vi "Utility MODBUS RTU CRC16.vi"(8 "error in (no error)":errorcluster, 10 "Message (empty array)":u8[](array[numeric]) format="%.0x", 11 "VISA resource name":refnum<visa-resource-name>) -> (0 "error out":errorcluster, 1 "CRC":u16 format="%.0x", 2 "Message with CRC":u8[](array[numeric]) format="%.0x", 3 "VISA resource name out":refnum<visa-resource-name>)   [LabVIEW 2010]
doc: "This VI computes the CRC code and appends it to the message."
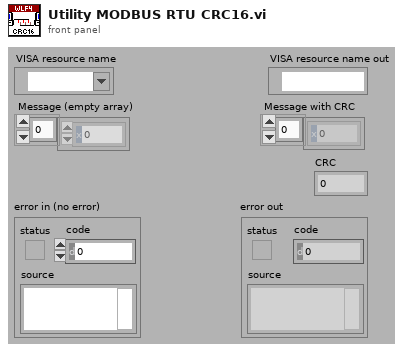
[diagram p1: front panel]
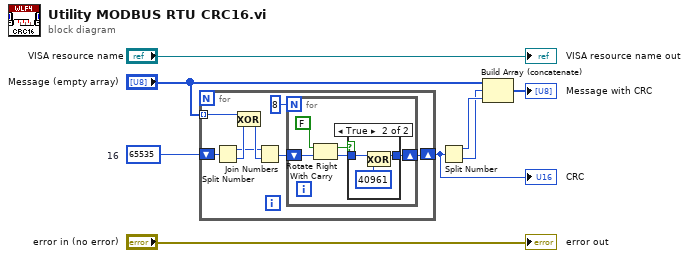
[diagram p0: block diagram]
diagram:
  w8 = u16 65535  # 16
  n1 = for {
    tunnel: "Message (empty array)" -> [w16] mode=indexing
    shift-right: [w9] -> w6
    shift-left: w8 -> [w14]
    n2 = Split Number(x=w14) -> (hi(x)=w11:u8, lo(x)=w13:u8)
    n3 = Exclusive Or(1:w13, 2:w16) -> (0:w12:u8)
    n4 = Join Numbers(hi=w11, lo=w12) -> ((hi.lo)=w10:u16)
    n5 = for {
      N: 8 -> [_]
      shift-right: [w17] -> w9
      shift-left: w10 -> [w21]
      n6 = Rotate Right With Carry(2:w21, 3:FALSE ("carry")) -> (0:w18:u16, 1:w19:bool)
      n7 = case shown="True" w19 {
        tunnel: w18 -> [w22 w25]
        tunnel: [w22 w23] -> w17
        frame False {
        }
        frame True {
          n8 = Exclusive Or(1:u16 40961 ("y"), 2:w25) -> (0:w23:u16)
        }
      }
    }
  }
  "CRC" <- w6
  n9 = Split Number(x=w6) -> (hi(x)=w5:u8, lo(x)=w4:u8)
  n10 = Build Array (concatenate)("Message (empty array)", w4, w5) -> (→"Message with CRC":u8[])
  "error out" <- "error in (no error)"
  "VISA resource name out" <- "VISA resource name"
